vi "Process-ICMP.vi"(9 "Frame":u8[](array[numeric])=[0, 80, 67, 160, 161, 162, 0, 35, 38, 182, 175, 53, 8, 0, 69, 0, 0, 60, 0, 8, 0, 0, 128, 1, 181, 215, 192, 168, 1, 200, 192, 168, 1, 201, 8, 0, 77, 90, 0, 1, 0, 1, 97, 98, 99, 100, 101, 102, 103, 104, 105, 106, 107, 108, 109, 110, 111, 112, 113, 114, 115, 116, 117, 118, 119, 97, 98, 99, 100, 101, 102, 103, 104, 105, 209, 148, 196, 117, 221] format="%02x") -> ()   [LabVIEW 2017]
panel:
  out "Header":T1
  out "ICMP Data":u8[](array[numeric])
  out "Protocol":u8=1
  out "IPv4 Payload":u8[](array[numeric])=[8, 0, 77, 90, 0, 1, 0, 1, 97, 98, 99, 100, 101, 102, 103, 104, 105, 106, 107, 108, 109, 110, 111, 112, 113, 114, 115, 116, 117, 118, 119, 97, 98, 99, 100, 101, 102, 103, 104, 105] format="%02x"
  # "Ethernet II"
  # "IPv4"
  # "ICMP"
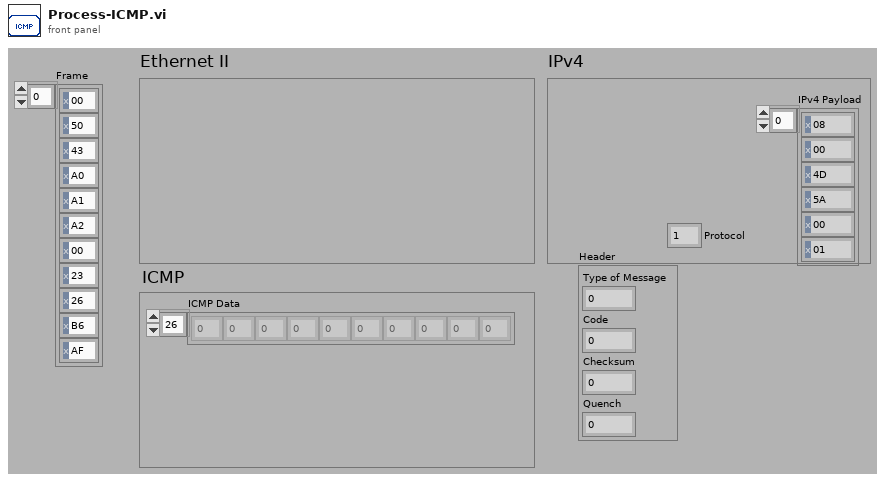
[diagram p1: front panel]
types:
  T1 = cluster{"Type of Message":u8, "Code":u8, "Checksum":u16, "Quench":u32}
  T2 = cluster{"Version":u8, "Header Length":u8, "Total Length":u16, "More Fragments":bool, "Don't Fragment":bool, "Fragment Offset":u16, "TTL":u8, "Header Checksum":u16, "Identification":u16, "Protocol":u8, "Source IP":u8[], "Destination IP":u8[]}
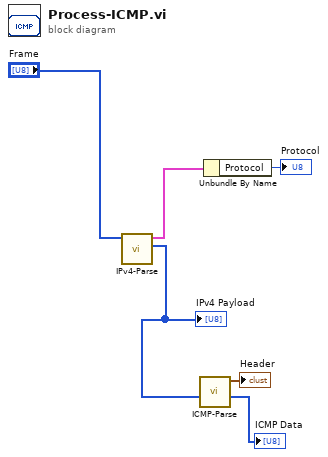
[diagram p0: block diagram]
diagram:
  n1 = call "IPv4-Parse.vi"("IPv4 Packet (in)"="Frame") -> ("IPv4 Payload"=w2:u8[], "Header"=w6:T2)  [unwired: 8 in, 1 out]
  "IPv4 Payload" <- w2
  n2 = call "ICMP-Parse.vi"("IPv4 Payload"=w2) -> ("Data"=→"ICMP Data":u8[], "Header"=→"Header":T1)  [unwired: 8 in, 1 out]
  n3 = Unbundle By Name(w6) -> ("Protocol"=→"Protocol":u8)
